vi "Get Scanner.vi"(8 "error in (no error)":errorcluster, 11 "Pulse Generator in":refnum<class "Pulse Generator.lvclass">) -> (0 "error out":errorcluster, 2 "Default Scanner out":refnum<class "Scanner.lvclass">)   [LabVIEW 2012, in "Pulse Generator.lvclass"]
doc: "(Dynamic) Returns the default Scanner object that scans over this Scannable. (Note that a Scannable may have multiple Scanners associated with it.) A Scanner is an analogue to an Iterator class in other languages."
uses:
  Pulse Generator.lvclass
  Scanners/Scanner/Scanner.lvclass
  LabVIEW-programs/Instruments/Utility Classes/Scannable/Scannable.lvclass
  Scanners/Pulse Gen Scan/Pulse Gen Scan.lvclass
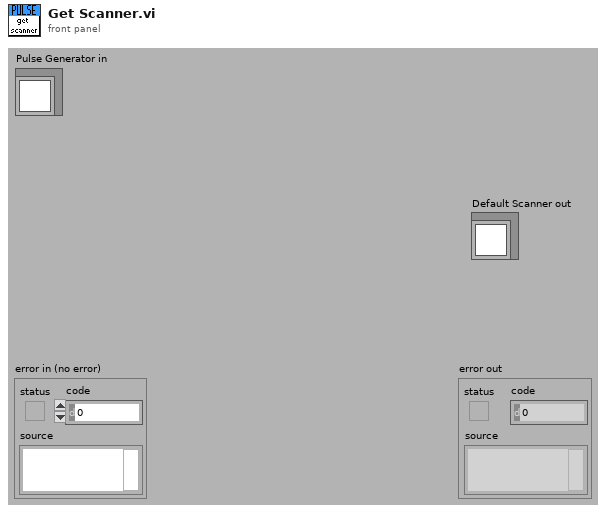
[diagram p1: front panel]
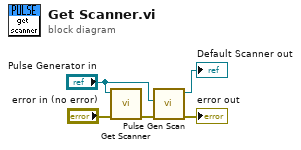
[diagram p0: block diagram]
diagram:
  n1 = call-parent "Get Scanner.vi"("error in (no error)"="error in (no error)", "Scannable in"="Pulse Generator in") -> ("error out"=w2:errorcluster)  [unwired: 9 out]
  n2 = call "Pulse Gen Scan.vi"("error in (no error)"=w2, "Pulse Generator.lvclass"="Pulse Generator in") -> ("error out"=→"error out":errorcluster, "Pulse Gen Scan out"=→"Default Scanner out":refnum<class "Pulse Gen Scan.lvclass">)  [unwired: 8 out]
